vi "Read State.vi"(8 "error in (no error)":errorcluster, 11 "AttackTacticVSS in":refnum<class "AttackTacticVSS.lvclass">) -> (0 "error out":errorcluster, 2 "State":enum16{"Kick", "Exit", "GoToBall", "BallToGoal"}(ring), 3 "AttackTacticVSS out":refnum<class "AttackTacticVSS.lvclass">)   [LabVIEW 2023, in "AttackTacticVSS.lvclass"]
uses:
  AttackTacticVSS.lvclass
  AttackTacticVSS.lvclass/AttackTacticVSS.ctl
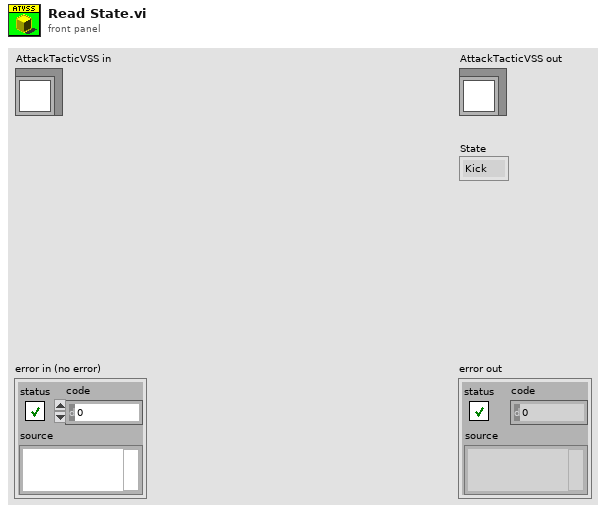
[diagram p1: front panel]
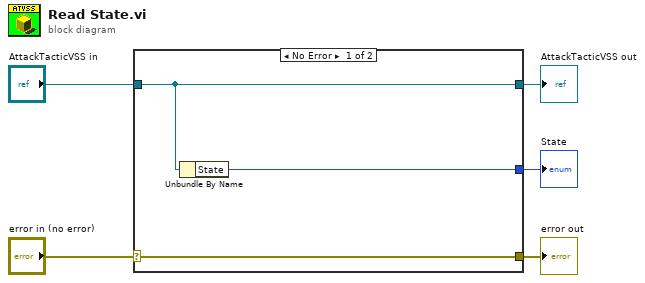
[diagram p0: block diagram]
diagram:
  n1 = case shown="No Error" "error in (no error)" {
    selector: "error in (no error)" -> [w8 w9]
    tunnel: [w8 w9] -> w4
    tunnel: [w7 w10] -> w2
    tunnel: "AttackTacticVSS in" -> [w7 w10]
    tunnel: [w6 _] -> w1
    frame No Error {
      n2 = Unbundle By Name(w7) -> ("State"=w6:enum16{"Kick", "Exit", "GoToBall", "BallToGoal"})
    }
    frame Error {
    }
  }
  "error out" <- w4
  "AttackTacticVSS out" <- w2
  "State" <- w1
